vi "close.vi"(8 "error in (no error)":errorcluster, 11 "16InOut in":refnum<class "16InOut.lvclass">) -> (0 "error out":errorcluster, 3 "16InOut out":refnum<class "16InOut.lvclass">)   [LabVIEW 2019, in "16InOut.lvclass"]
uses:
  16InOut.lvclass
  IOCard.lvclass
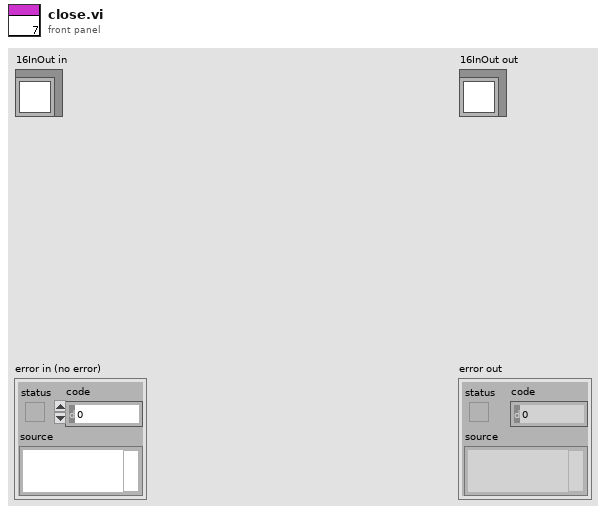
[diagram p1: front panel]
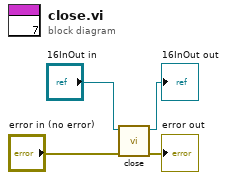
[diagram p0: block diagram]
diagram:
  n1 = call-parent "close.vi"("error in (no error)"="error in (no error)", "IOCard in"="16InOut in") -> ("error out"=→"error out":errorcluster, "IOCard out"=→"16InOut out":refnum<class "16InOut.lvclass">)  [unwired: 8 in]
